vi "read_script.vi"(8 "error in (no error)":errorcluster caption="entrée d'erreur (pas d'erreur)", 11 "Model en entrée":refnum<class "Model.lvclass">) -> (0 "error out":errorcluster caption="sortie d'erreur", 2 "script":string="import sys\nimport numpy as np\nimport joblib\nimport scipy\nimport json\n\nmemory={}\nout=['ok']\n\ndef init_model(params):\n    global memory\n    {import}\n    memory['model'] = {model}(**(json.loads(params)))\n\ndef set_params(params):\n    global memory\n    params = json.loads(params)\n    memory['model'].set_params(**params)\n\ndef get_params():\n    global memory\n    params = memory['model'].get_params()\n    params = special_case(params)\n    return json.dumps(params)\n\ndef get_attributes(attributes_needed):\n    names = json.loads(attributes_needed).keys()\n    attributes = {key:value for key,value in memory['model'].__dict__.items() if key in names}\n    attributes = special_case(attributes)\n    return json.dumps(attributes)\n\ndef fit(data):\n    data = json.loads(data)\n    import inspect\n    data_needed = list(inspect.signature(memory['model'].fit).parameters)\n    correct_data = {key:data[key] for key in data_needed if (key in data.keys() and len(data[key])>0)}\n    memory['model'].fit(**correct_data)\n\ndef special_case(d):\n    for key in d.keys():\n        if str(type(d[key]))==\"<class 'function'>\": d[key] = d[key].__name__\n        if str(type(d[key]))==\"<class 'numpy.ndarray'>\": d[key] = d[key].tolist()\n    return d\n\ndef exec_code(code):\n    global memory\n    global out\n    try:\n        exec(code)\n        if type(out[0]) == np.ndarray:\n            out[0] = out[0].tolist()\n        elif type(out[0]) == scipy.sparse.csr.csr_matrix:\n            out[0] = out[0].tocoo()\n            out[0] = list(zip(out[0].row, out[0].col, out[0].data))\n        return str(out)\n    except:\n        erreur = sys.exc_info()\n        typerr = u\"%s\" % (erreur[0])\n        typerr = typerr[typerr.find(\"'\")+1:typerr.rfind(\"'\")]\n        msgerr = u\"%s\" % (erreur[1])\n        message = str('/!\\\\ {0} : {1}'. format(typerr,msgerr))\n        return message \n    \n\ndef save_model(UserModelName=str,path=str,Save_name=str):\n    try:\n        filename=path+'\\{}.gz'.format(Save_name)\n        joblib.dump(memory[UserModelName],filename=filename)\n        return filename\n    except:\n        erreur = sys.exc_info()\n        typerr = u\"%s\" % (erreur[0])\n        typerr = typerr[typerr.find(\"'\")+1:typerr.rfind(\"'\")]\n        msgerr = u\"%s\" % (erreur[1])\n        message = str('/!\\\\ {0} : {1}'. format(typerr,msgerr))\n        return message \n    \n\ndef load_model(UserModelName=str,file=str):\n\n    try:\n        memory[UserModelName]=joblib.load(filename=file) \n        return str(memory[UserModelName])\n    except:\n        erreur = sys.exc_info()\n        typerr = u\"%s\" % (erreur[0])\n        typerr = typerr[typerr.find(\"'\")+1:typerr.rfind(\"'\")]\n        msgerr = u\"%s\" % (erreur[1])\n        message = str('/!\\\\ {0} : {1}'. format(typerr,msgerr))\n        return message\n    \ndef get_help(UserModelName=str):\n    try:\n        return str(memory[UserModelName].__doc__)\n    except:\n        erreur = sys.exc_info()\n        typerr = u\"%s\" % (erreur[0])\n        typerr = typerr[typerr.find(\"'\")+1:typerr.rfind(\"'\")]\n        msgerr = u\"%s\" % (erreur[1])\n        message = str('/!\\\\ {0} : {1}'. format(typerr,msgerr))\n        return message \n    ", 3 "Model en sortie":refnum<class "Model.lvclass">)   [LabVIEW 2020, in "Model.lvclass"]
uses:
  Model.lvclass
  Model.lvclass/Model.ctl
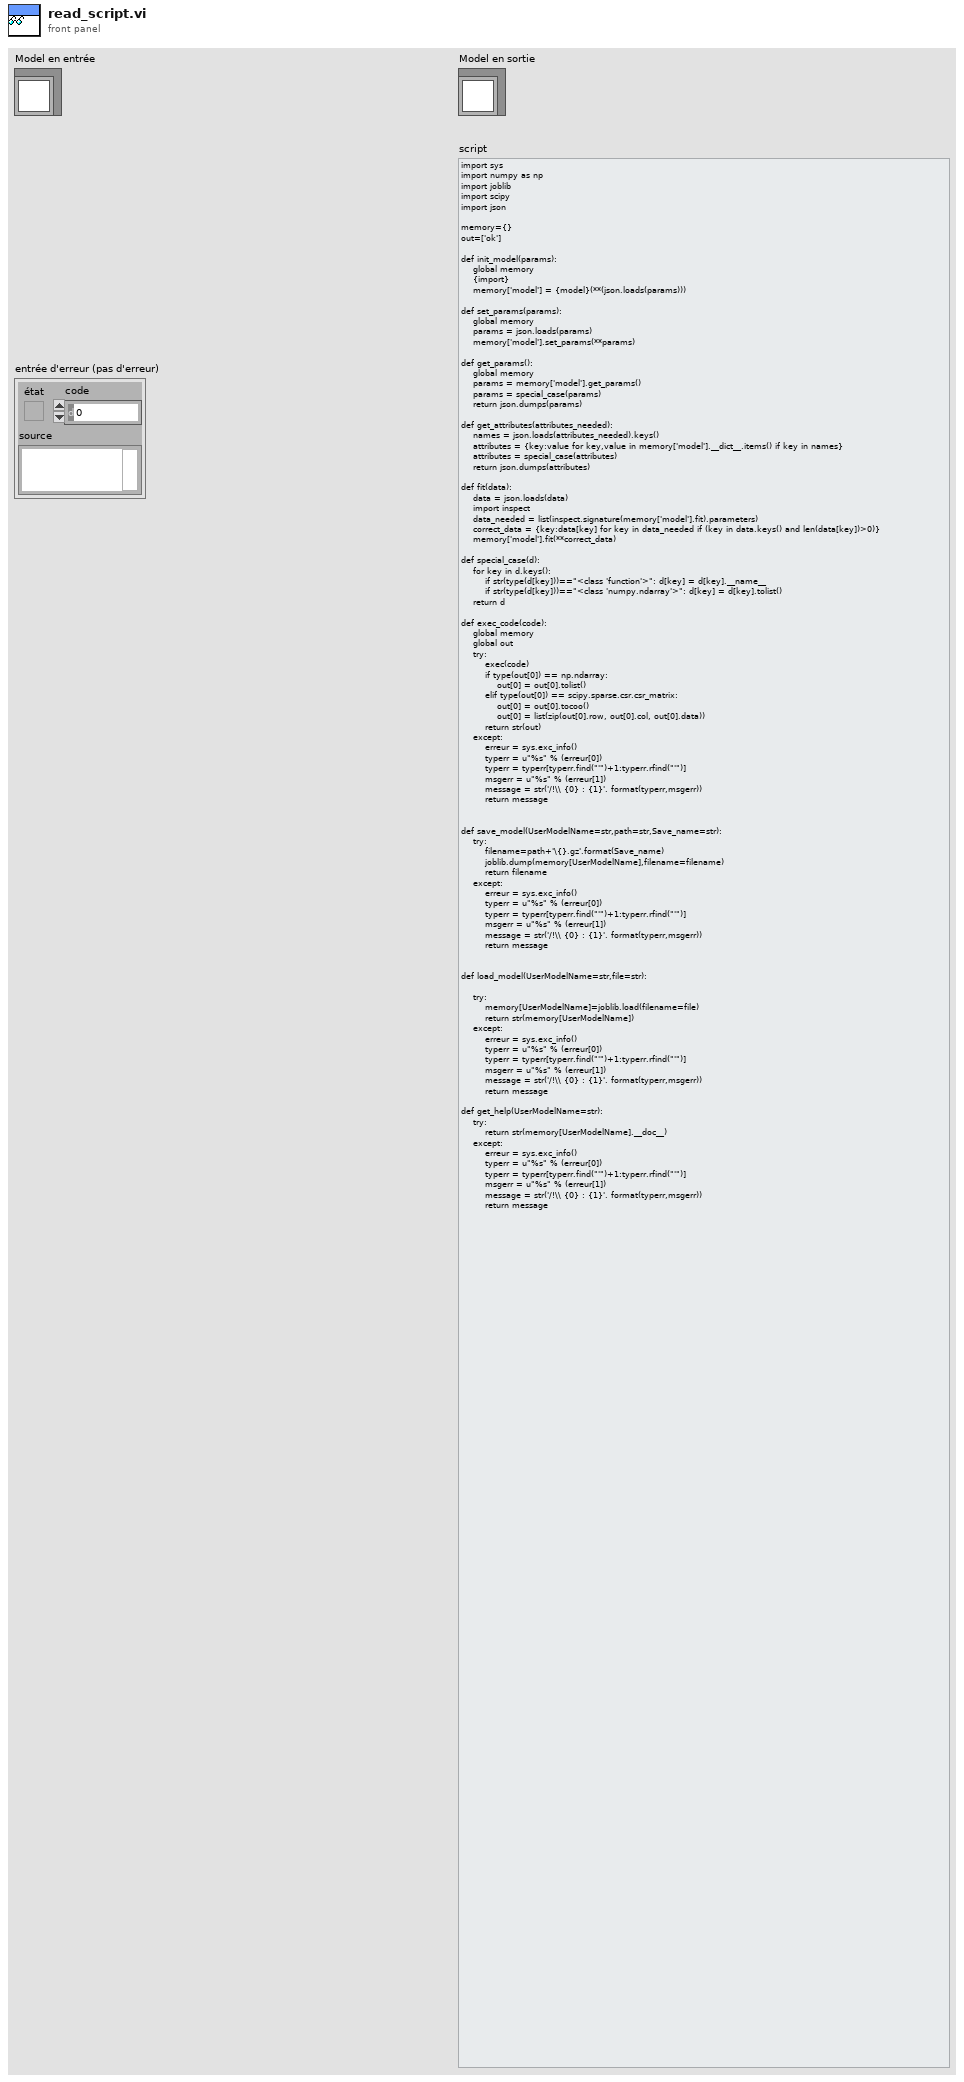
[diagram p1: front panel]
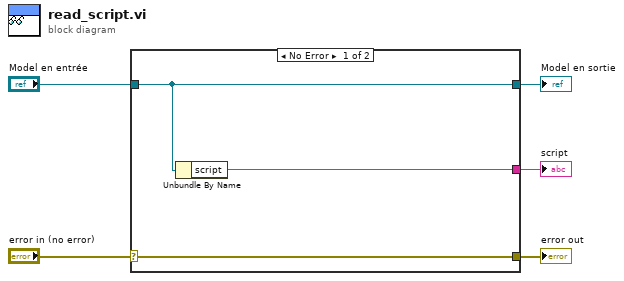
[diagram p0: block diagram]
diagram:
  n1 = case shown="No Error" "error in (no error)" {
    selector: "error in (no error)" -> [w8 w9]
    tunnel: [w8 w9] -> w4
    tunnel: [w7 w10] -> w2
    tunnel: "Model en entrée" -> [w7 w10]
    tunnel: [w6 _] -> w1
    frame No Error {
      n2 = Unbundle By Name(w7) -> ("script"=w6:string)
    }
    frame Error {
    }
  }
  "error out" <- w4
  "Model en sortie" <- w2
  "script" <- w1
